vi "Tool ID holder slaves.vi"(1 "Action(GET)":enum16{"GET", "SET"}(ring), 5 "Set index":i32, 7 "value in":T1[](array[typedef]) {"LEIN implementation code" format="%.0x"; "Serial number" format="%04.0f"; "HW REV" format="%02x"}, 11 "error in (no error)":errorcluster) -> (8 "value out":T1[](array[typedef]) {"LEIN implementation code" format="%.0x"; "Serial number" format="%04.0f"; "HW REV" format="%02x"}, 15 "error out":errorcluster)   [LabVIEW 2011]
uses:
  LEINmaster/Defenitions/LEIN STAT 15 Id system cluster v2 wo lables.ctl
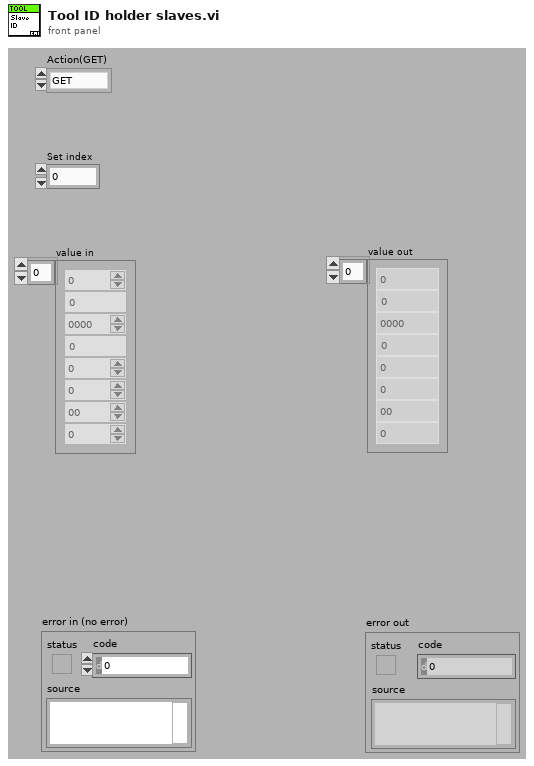
[diagram p1: front panel]
types:
  T1 = typedef "LEIN STAT 15 Id system cluster v2 wo lables.ctl" = cluster{"LEIN version":u8, "LEIN implementation code":u8, "Serial number":u16, "Project":u16, "HW ID":u8, "FW ID":u8, "HW REV":u8, "FW REV":u8}
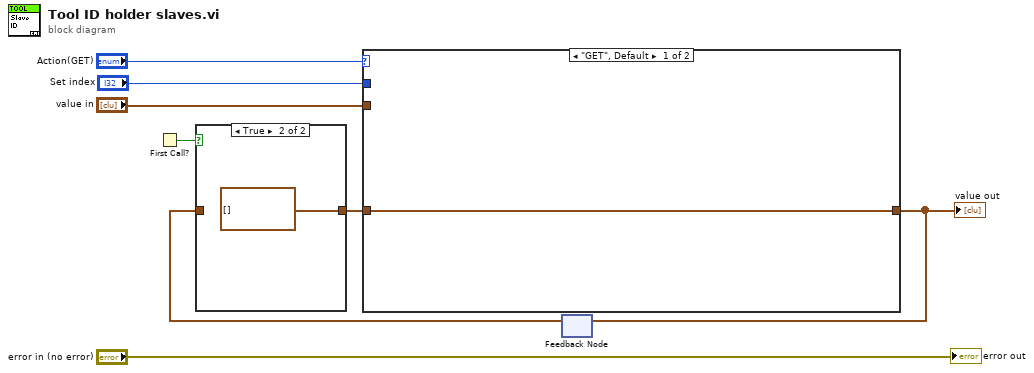
[diagram p0: block diagram]
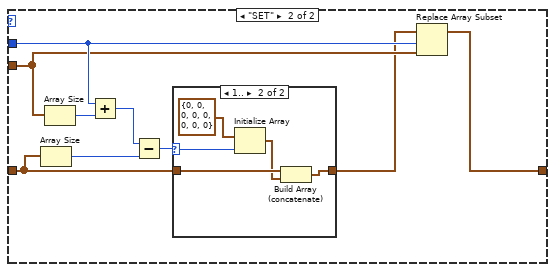
[diagram p3: hidden frame]
diagram:
  n1 = First Call?() -> (First Call?: T/F=w5:bool)
  n2 = feedback #1() -> (w6:T1[])  [unwired: 1 in]
  n3 = case shown="True" w5 {
    tunnel: w6 -> [w9 _]
    tunnel: [w9 T1[] [] ("value")] -> w3
    frame False {
    }
    frame True {
    }
  }
  n4 = case shown="\"GET\", Default" "Action(GET)" {
    tunnel: [w11 w12] -> w4
    tunnel: w3 -> [w11 w17]
    tunnel: "value in" -> [_ w14]
    tunnel: "Set index" -> [_ w15]
    frame "GET", Default {
    }
    frame "SET" {
      n5 = Array Size(array=w17) -> (size(s)=w18:i32)
      n6 = Array Size(array=w14) -> (size(s)=w20:i32)
      n7 = Add(x=w15, y=w20) -> (x+y=w19:i32)
      n8 = Subtract(x=w19, y=w18) -> (x-y=w16:i32)
      n9 = case shown="1.." w16 {
        selector: w16 -> [_ w26]
        tunnel: w17 -> [w21 w24]
        tunnel: [w21 w22] -> w13
        frame 0, Default {
        }
        frame 1.. {
          n10 = Initialize Array(T1 {"LEIN version"=0, "LEIN implementation code"=0, "Serial number"=0, "Project"=0, "HW ID"=0, "FW ID"=0, "HW REV"=0, "FW REV"=0} ("Solenoid"), w26) -> (w23:T1[])
          n11 = Build Array (concatenate)(w24, w23) -> (w22:T1[])
        }
      }
      n12 = Replace Array Subset(array=w13, new element=w14, index=w15) -> (w12:T1[])
    }
  }
  "value out" <- w4
  n13 = feedback-in #1(w4) -> ()
  "error out" <- "error in (no error)"
